vi "Load External Modules.vi"(8 "error in (no error)":errorcluster, 11 "Application Controller in":refnum<class "Application Controller.lvclass">) -> (0 "error out":errorcluster, 3 "Application Controller out":refnum<class "Application Controller.lvclass">)   [LabVIEW 2020, in "Application Controller.lvclass"]
uses:
  Application Controller.lvclass
  Application Controller.lvclass/Application Controller.ctl
  Template Module/Template Module.lvclass/Template Module.ctl
  Template Module/Read Name.vi
  Read Start-up configuration file.vi
  Template Module/Template Module.lvclass
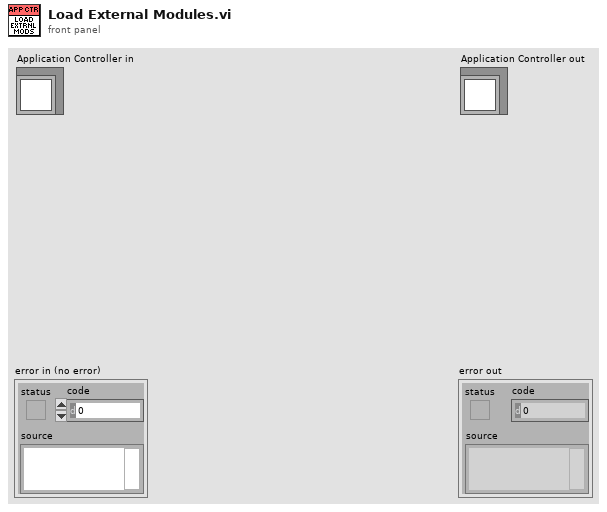
[diagram p1: front panel]
types:
  T1 = typedef "Menu Control.ctl" = enum16{"NONE", "Monitor", "Post-process", "Pulse"}
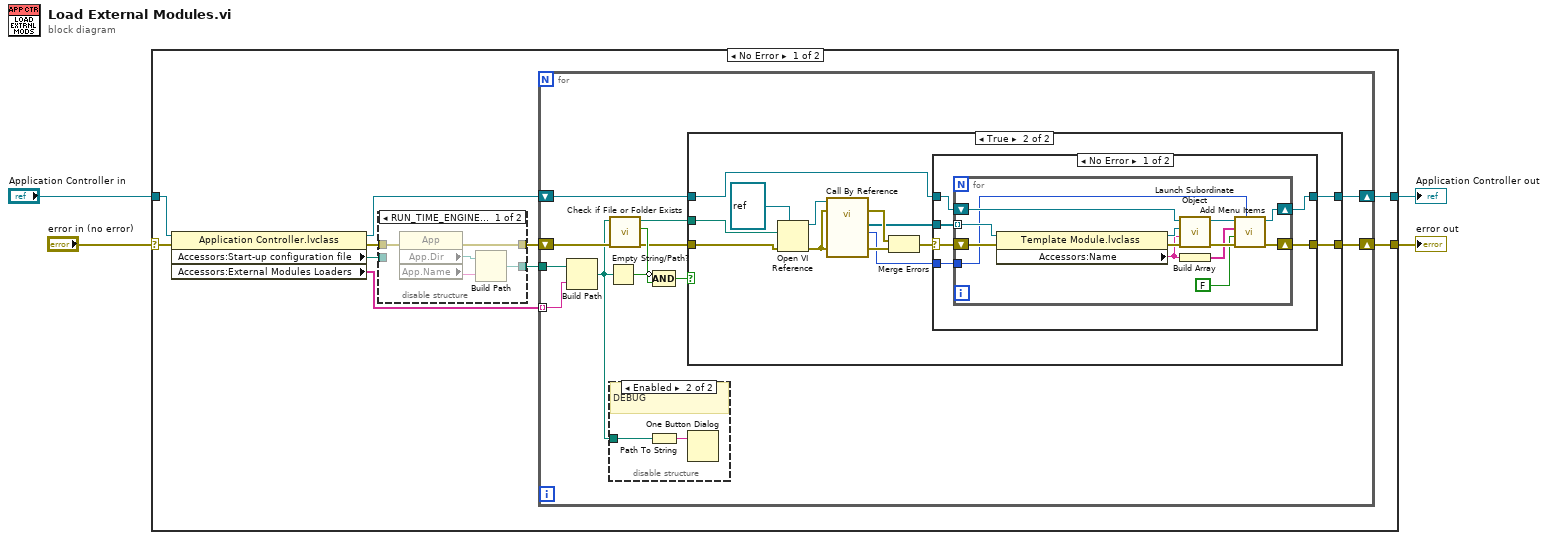
[diagram p0: block diagram]
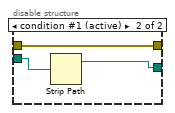
[diagram p2: hidden frame]
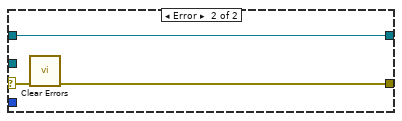
[diagram p5: hidden frame]
diagram:
  n1 = case shown="No Error" "error in (no error)" {
    selector: "error in (no error)" -> [w14 w75]
    tunnel: [w12 w75] -> w3
    tunnel: [w10 w74] -> w1
    tunnel: "Application Controller in" -> [w13 w74]
    frame No Error {
      n2 = property class="Application Controller.lvclass"(reference=w13, error in=w14) -> (reference out=w11:refnum<class "Application Controller.lvclass">, error out=w7:errorcluster, "Accessors:Start-up configuration file"=w9:path, "Accessors:External Modules Loaders"=w5:string[])
      n3 = disable-structure shown="RUN_TIME_ENGINE==True, Default" {
        disable-tunnel: w9 -> [_ w22]
        disable-tunnel: [w15 w21] -> w8
        disable-tunnel: w7 -> [w19 w20]
        disable-tunnel: [w18 w20] -> w6
        frame condition #0 {
          n4 = property class="App"(error in=w19) -> (error out=w18:errorcluster, "App.Dir"=w17:path, "App.Name"=w16:string)  [unwired: 1 in, 1 out]
          n5 = Build Path(base path=w17, name or relative path=w16) -> (appended path=w15:path)
        }
        frame condition #1 (active) {
          n6 = Strip Path(path=w22) -> (stripped path=w21:path)  [unwired: 1 out]
        }
      }
      n7 = for {
        tunnel: w5 -> [w24] mode=indexing
        shift-right: [w27] -> w12
        shift-left: w6 -> [w32]
        shift-right: [w26] -> w10
        shift-left: w11 -> [w28]
        tunnel: w8 -> [w25]
        n8 = Build Path(base path=w25, name or relative path=w24) -> (appended path=w23:path)
        n9 = Empty String/Path?(string/path=w23) -> (empty?=w34:bool)
        n10 = call <vilib>:"Check if File or Folder Exists.vi"("error in (no error)"=w32, "path"=w23) -> ("error out"=w30:errorcluster, "file or folder exists?"=w33:bool, "dup path"=w29:path)  [unwired: 7 in]
        n11 = disable-structure shown="Enabled" {
          disable-tunnel: w23 -> [_ w36]
          frame Disabled {
          }
          frame Enabled {
            # "DEBUG"
            n12 = Path To String(path=w36) -> (string=w35:string)
            n13 = One Button Dialog(message=w35) -> ()  [unwired: 1 in, 1 out]
          }
        }
        n14 = Compound Arithmetic op=AND(invert w34, w33) -> (w31:bool)
        n15 = case shown="True" w31 {
          tunnel: w30 -> [w38 w49]
          tunnel: w29 -> [_ w48]
          tunnel: w28 -> [w37 w43]
          tunnel: [w38 w41] -> w27
          tunnel: [w37 w40] -> w26
          frame False {
          }
          frame True {
            n16 = Open VI Reference(type specifier VI Refnum (for type only)=refnum<vi> refnum, vi path=w48, error in (no error)=w49) -> (vi reference=w51:refnum<vi>, error out=w47:errorcluster)  [unwired: 3 in]
            n17 = call-by-ref "?"(reference=w51, error in=w47, "Error In"=w47) -> (error out=w46:errorcluster, "Error Out"=w45:errorcluster, "Menu control"=w39:T1, "Modules"=w42:refnum<class "Template Module.lvclass">[])  [unwired: 8 in, 1 out]
            n18 = Merge Errors(w46, w45) -> (w44:errorcluster)
            n19 = case shown="No Error" w44 {
              selector: w44 -> [w56 w73]
              tunnel: w43 -> [w55 w71]
              tunnel: w42 -> [w57 _]
              tunnel: [w54 w72] -> w41
              tunnel: [w53 w71] -> w40
              tunnel: w39 -> [w52 _]
              frame No Error {
                n20 = for {
                  tunnel: w57 -> [w70] mode=indexing
                  shift-right: [w59] -> w53
                  shift-left: w55 -> [w66]
                  shift-right: [w60] -> w54
                  shift-left: w56 -> [w69]
                  tunnel: w52 -> [w58]
                  n21 = property class="Template Module.lvclass"(reference=w70, error in=w69) -> (reference out=w67:refnum<class "Template Module.lvclass">, error out=w68:errorcluster, "Accessors:Name"=w63:string)
                  n22 = call-dynamic "Launch Subordinate Object.vi"("error in (no error)"=w68, "Name"=w63, "Subordinate Object"=w67, "Application Controller in"=w66) -> ("error out"=w64:errorcluster, "Application Controller out"=w65:refnum<class "Application Controller.lvclass">)  [unwired: 5 in, 1 out]
                  n23 = Build Array(w63) -> (w62:string[])
                  n24 = call-dynamic "Add Menu Items.vi"("Menu control"=w58, "error in (no error)"=w64, "Reset"=FALSE, "Item Names"=w62, "Application Controller in"=w65) -> ("error out"=w60:errorcluster, "Application Controller out"=w59:refnum<class "Application Controller.lvclass">)  [unwired: 5 in]
                }
              }
              frame Error {
                n25 = call <vilib>:"Clear Errors.vi"("error in (no error)"=w73) -> ("error out"=w72:errorcluster)  [unwired: 5 in, 1 out]
              }
            }
          }
        }
      }
    }
    frame Error {
    }
  }
  "error out" <- w3
  "Application Controller out" <- w1
